vi "PC_DCG to DPWMM.vi"() -> ()   [LabVIEW 2021]
uses:
  Digital Clock Generation/Typedefs/Digital Clock Settings.ctl
  Digital Clock Generation/Typedefs/Actual Clock Settings.ctl
  Digital PWM Measurement/Typedefs/Digital PWM Measurements.ctl
  Common/Typedefs/Execution Options - Measure.ctl
  Digital PWM Measurement/DAQ_Digital PWM Measurement.lvlib
  Digital Clock Generation/DAQ_Digital Clock Generation.lvlib
panel:
  out "Actual Cycles Captured":i32=2
  out "Digital PWM Measurements":T1={"High Time (s)"=5e-05, "Low Time (s)"=5e-05, "Duty Cycle (%)"=50.0, "Frequency (Hz)"=10000.0} {"Frequency (Hz)" format="%.6p"; "Duty Cycle (%)" min=0.0 max=100.0 format="%#.2p"; "Low Time (s)" format="%.2p"; "High Time (s)" format="%.2p"}
  out "error out":errorcluster
  in  "Cycles to capture":i32=2 min=2 step=1
  out "Actual Clock Settings":T2={"Frequency (Hz)"=10000.0, "Duty Cycle (%)"=50.0, "Generation Time (s)"=0.1} {"Duty Cycle (%)" format="%#.2p"; "Frequency (Hz)" format="%.6p"; "Generation Time (s)" format="%.2p"}
  in  "Digital Clock Settings":T3={"Frequency (Hz)"=10000.0, "Duty Cycle(%)"=50.0, "Generation Time (s)"=0.1} {"Duty Cycle(%)" format="%#.2p"; "Frequency (Hz)" format="%.6p"; "Generation Time (s)" format="%.2p"}
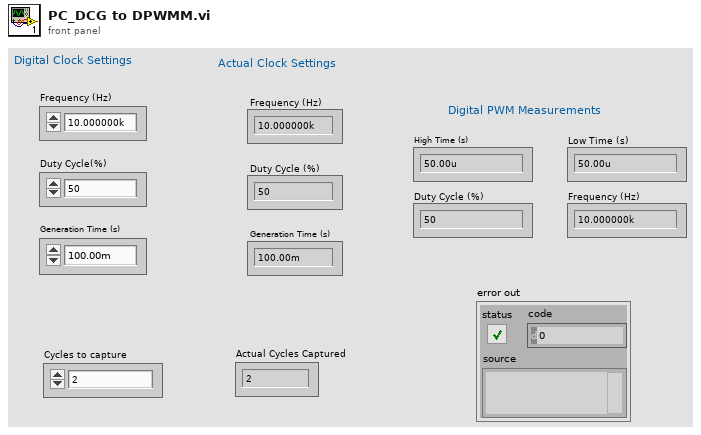
[diagram p1: front panel]
types:
  T1 = typedef "DAQ_Digital PWM Measurement.lvlib/Digital PWM Measurements.ctl" = cluster{"High Time (s)":dbl, "Low Time (s)":dbl, "Duty Cycle (%)":dbl, "Frequency (Hz)":dbl}
  T2 = typedef "DAQ_Digital Clock Generation.lvlib/Actual Clock Settings.ctl" = cluster{"Frequency (Hz)":dbl, "Duty Cycle (%)":dbl, "Generation Time (s)":dbl}
  T3 = typedef "DAQ_Digital Clock Generation.lvlib/Digital Clock Settings.ctl" = cluster{"Frequency (Hz)":dbl, "Duty Cycle(%)":dbl, "Generation Time (s)":dbl}
  T4 = typedef "Execution Options - Measure.ctl" = enum16{"Configure & Measure", "Configure only", "Measure only"}
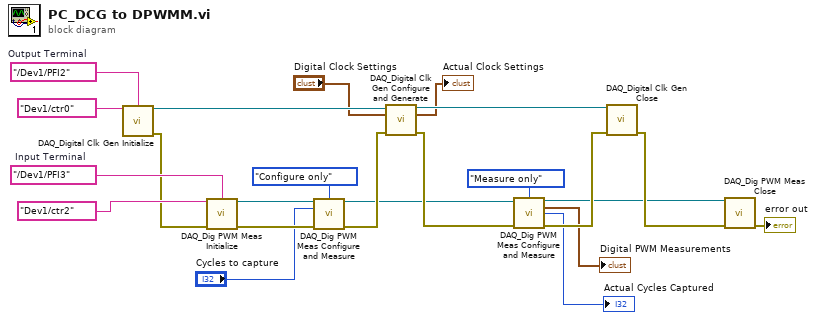
[diagram p0: block diagram]
diagram:
  w22 = tag "/Dev1/PFI2"  # Output Terminal
  w21 = tag "/Dev1/PFI3"  # Input Terminal
  n1 = call "DAQ_Digital Clk Gen Initialize.vi"("Physical Channel (Counter)"=tag "Dev1/ctr0", "Output Terminal"=w22) -> ("DAQmx Task Out"=w12:refnum<k21>, "error out"=w19:errorcluster)  [unwired: 12 in]
  n2 = call "DAQ_Dig PWM Meas Initialize.vi"("Physical Channel (counter)"=tag "Dev1/ctr2", "Input Terminal"=w21, "error in"=w19) -> ("DAQmx Task Out"=w18:refnum<k21>, "error out"=w17:errorcluster)  [unwired: 11 in]
  n3 = call "DAQ_Dig PWM Meas Configure and Measure.vi"("DAQmx Task In"=w18, "Execution Option"=Execution_Options_-_Measure."Configure only", "Cycles to capture"="Cycles to capture", "error in"=w17) -> ("DAQmx Task Out"=w10:refnum<k21>, "error out"=w16:errorcluster)  [unwired: 8 in, 2 out]
  n4 = call "DAQ_Digital Clk Gen Configure and Generate.vi"("DAQmx Task In"=w12, "Digital Clock Settings"="Digital Clock Settings", "error in"=w16) -> ("DAQmx Task Out"=w11:refnum<k21>, "Actual Clock Settings"=→"Actual Clock Settings":T2, "error out"=w15:errorcluster)  [unwired: 10 in]
  n5 = call "DAQ_Dig PWM Meas Configure and Measure.vi"("DAQmx Task In"=w10, "Execution Option"=Execution_Options_-_Measure."Measure only", "error in"=w15) -> ("DAQmx Task Out"=w9:refnum<k21>, "Digital PWM Measurements"=→"Digital PWM Measurements":T1, "Actual Cycles Captured"=→"Actual Cycles Captured":i32, "error out"=w14:errorcluster)  [unwired: 9 in]
  n6 = call "DAQ_Digital Clk Gen Close.vi"("DAQmx Task In"=w11, "error in"=w14) -> ("error out"=w13:errorcluster)  [unwired: 13 in]
  n7 = call "DAQ_Dig PWM Meas Close.vi"("DAQmx Task In"=w9, "error in"=w13) -> ("error out"=→"error out":errorcluster)  [unwired: 13 in]
